vi "SISO_LOOPBACK.vi"() -> ()   [LabVIEW 2012]
panel:
  out "Constellation":cluster{dbl[], dbl[]}[](graph)
  in  "Channel conf":T1={"Atenuation [dB]"=6.0, "Noise Std. Dev."=0.0, "Initial phase [deg]"=125.0, "Freq. Shift [Hz/Hz]"=0.001} {"Freq. Shift [Hz/Hz]" min=0.0 max=1.0 step=0.0001 format="%0.4f"; "Noise Std. Dev." format="%0.2f"; "Atenuation [dB]" format="%0.2f"}
  out "Rx data":string[](array[string])=["The quick brown fox jumps over the lazy dog", "El veloz murciélago hindú comía feliz cardillo y kiwi", "Jove xef, porti whisky amb quinze glaçons d'hidrogen, coi!", ""]
  out "Link occupation [%]":dbl(knob)=25.87890625 scale=0.0..100.0
  in  "Tx data":string[](array[string])=["The quick brown fox jumps over the lazy dog", "El veloz murciélago hindú comía feliz cardillo y kiwi", "Jove xef, porti whisky amb quinze glaçons d'hidrogen, coi!"]
  in  "System options":T2={"Samples per symbol"=6, "Roll-Off"=0.75, "Filter length (symbols)"=3, "Symbols/Pilot"=8, "Modulation Type"=enum."64-QAM", "Payload Symbols"=1024} {"Payload Symbols" min=32 max=8192 step=16; "Symbols/Pilot" min=6 max=16 step=2; "Filter length (symbols)" min=1 max=9 step=2; "Roll-Off" min=0.0 max=1.0 step=0.01; "Samples per symbol" min=2 max=32 step=2}
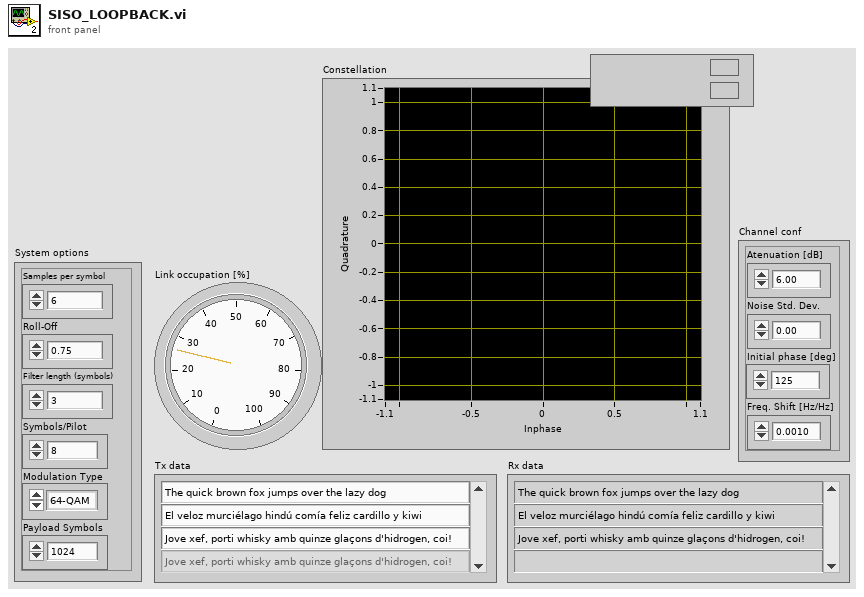
[diagram p1: front panel]
types:
  T1 = cluster{"Atenuation [dB]":dbl, "Noise Std. Dev.":dbl, "Initial phase [deg]":dbl, "Freq. Shift [Hz/Hz]":dbl}
  T2 = cluster{"Samples per symbol":i32, "Roll-Off":dbl, "Filter length (symbols)":i32, "Symbols/Pilot":i32, "Modulation Type":enum16{"BPSK", "4-QAM", "16-QAM", "64-QAM"}, "Payload Symbols":i32}
  T3 = cluster{"Samples per symbol":i32, "Roll-Off":dbl, "Filter length (symbols)":i32}
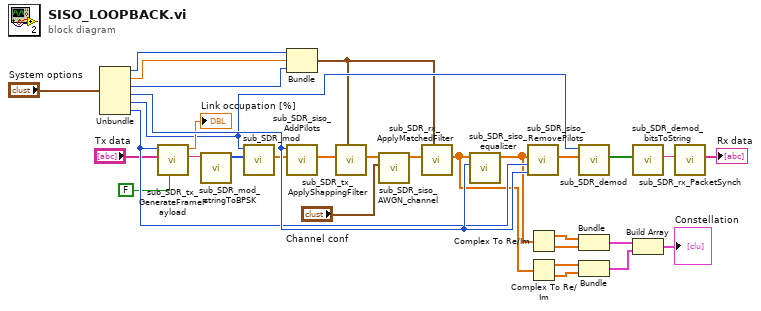
[diagram p0: block diagram]
diagram:
  n1 = Unbundle("System options") -> ("Samples per symbol"=w18:i32, "Roll-Off"=w17:dbl, "Filter length (symbols)"=w16:i32, "Symbols/Pilot"=w30:i32, "Modulation Type"=w22:enum16{"BPSK", "4-QAM", "16-QAM", "64-QAM"}, "Payload Symbols"=w27:i32)
  n2 = call "sub_SDR_tx_GenerateFramePayload.vi"("Init?"=FALSE, "Packets"="Tx data", "Payload Length"=w27) -> ("Payload String"=w28:string, "Link occupation [%]"=→"Link occupation [%]":dbl)  [unwired: 6 in, 1 out]
  n3 = call "sub_SDR_mod_stringToBPSK.vi"("Input String"=w28) -> ("Array"=w29:i16[])  [unwired: 10 in]
  n4 = call "sub_SDR_mod.vi"("Array"=w29, "Modulation Type"=w22) -> ("Array out"=w21:cdb[])  [unwired: 9 in]
  n5 = Bundle("Samples per symbol"=w18, "Roll-Off"=w17, "Filter length (symbols)"=w16) -> (w19:T3)  [unwired: 1 in]
  n6 = call "sub_SDR_siso_AddPilots.vi"("Array in"=w21, "Symbols/Pilots"=w30) -> ("Array Out"=w20:cdb[])  [unwired: 9 in]
  n7 = call "sub_SDR_tx_ApplyShappingFilter.vi"("Filter Options"=w19, "Data Symbols"=w20) -> ("Shaped symbols"=w12:cdb[])  [unwired: 9 in]
  n8 = call "sub_SDR_siso_AWGN_channel.vi"("Channel conf"="Channel conf", "Channel In"=w12) -> ("Channel Out"=w11:cdb[])  [unwired: 9 in]
  n9 = call "sub_SDR_rx_ApplyMatchedFilter.vi"("Filter Options"=w19, "Received stream"=w11) -> ("Received Symbols"=w1:cdb[])  [unwired: 9 in]
  n10 = call "sub_SDR_siso_equalizer.vi"("Symbols/Pilot"=w30, "In frame"=w1) -> ("Out Frame"=w2:cdb[])  [unwired: 9 in]
  n11 = call "sub_SDR_siso_RemovePilots.vi"("Symbols per pilot"=w30, "Payload Symbols"=w27, "Array in"=w2) -> ("Array Out"=w23:cdb[])  [unwired: 7 in, 1 out]
  n12 = Complex To Re/Im(x + iy=w2) -> (x=w8:dbl[], y=w9:dbl[])
  n13 = Complex To Re/Im(x + iy=w1) -> (x=w7:dbl[], y=w6:dbl[])
  n14 = call "sub_SDR_demod.vi"("Input Symbols"=w23, "Modulation Type"=w22) -> ("Output bits"=w15:bool[])  [unwired: 8 in, 1 out]
  n15 = Bundle(w8, w9) -> (w5:cluster{dbl[], dbl[]})  [unwired: 1 in]
  n16 = Bundle(w7, w6) -> (w4:cluster{dbl[], dbl[]})  [unwired: 1 in]
  n17 = call "sub_SDR_demod_bitsToString.vi"("Input bits"=w15) -> ("Output string"=w14:string)  [unwired: 10 in]
  n18 = Build Array(w5, w4) -> (→"Constellation":cluster{dbl[], dbl[]}[])
  n19 = call "sub_SDR_rx_PacketSynch.vi"("Input Stream"=w14) -> ("Output Packets"=→"Rx data":string[])  [unwired: 9 in, 1 out]
